vi "ping connection and reopen if needed.vi"(8 "error in (no error)":errorcluster, 11 "mysql in":refnum<class "mysql.lvclass">) -> (0 "error out":errorcluster, 3 "mysql out":refnum<class "mysql.lvclass">)   [LabVIEW 2020, in "mysql.lvlib" / "mysql.lvclass"]
uses:
  mysql.lvclass
  mysql.lvclass/mysql.ctl
  MySql.Data
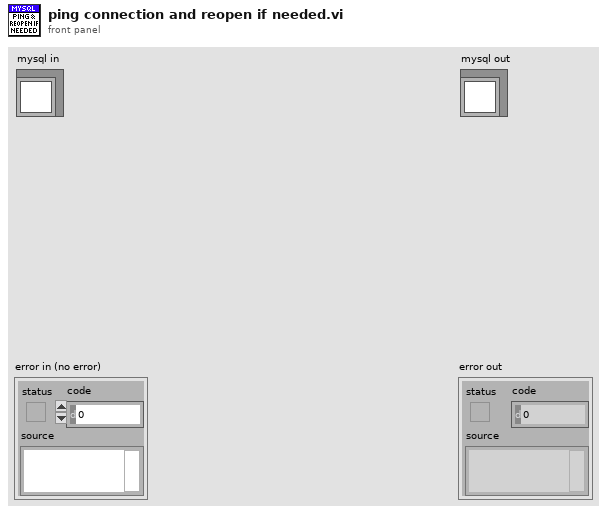
[diagram p1: front panel]
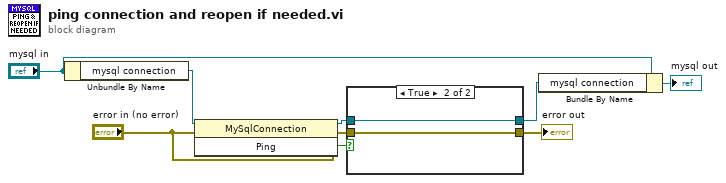
[diagram p0: block diagram]
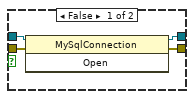
[diagram p2: hidden frame]
diagram:
  n1 = Unbundle By Name("mysql in") -> ("mysql connection"=w8:refnum<k24>)
  n2 = invoke class="MySqlConnection" method="Ping"(reference=w8, error in="error in (no error)") -> (reference out=w7:refnum<k24>, "Ping"=w6:bool)  [unwired: 1 in, 1 out]
  n3 = case shown="True" w6 {
    tunnel: w7 -> [w12 w13]
    tunnel: "error in (no error)" -> [w11 w14]
    tunnel: [w9 w14] -> w5
    tunnel: [w10 w13] -> w2
    frame False {
      n4 = invoke class="MySqlConnection" method="Open"(reference=w12, error in=w11) -> (reference out=w10:refnum<k24>, error out=w9:errorcluster)  [unwired: 1 in, 1 out]
    }
    frame True {
    }
  }
  "error out" <- w5
  n5 = Bundle By Name(cluster="mysql in", "mysql connection"=w2) -> (→"mysql out":refnum<class "mysql.lvclass">)
